vi "Variant to String.vi"(8 "error in (no error)":errorcluster, 10 "Variant":variant, 11 "Integer Value in":refnum<class "Integer Value.lvclass">) -> (0 "error out":errorcluster, 2 "String":string, 3 "Integer Value out":refnum<class "Integer Value.lvclass">)   [LabVIEW 2020, in "Composed Columns.lvlib" / "Integer Value.lvclass"]
uses:
  Integer Value.lvclass
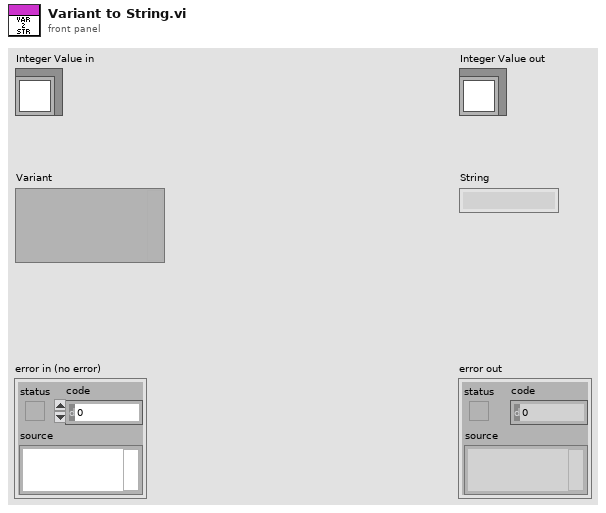
[diagram p1: front panel]
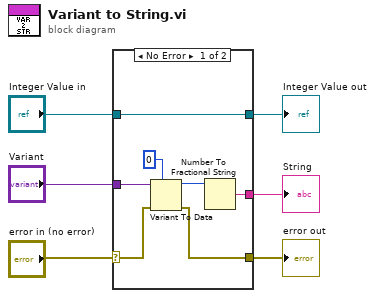
[diagram p0: block diagram]
diagram:
  n1 = case shown="No Error" "error in (no error)" {
    selector: "error in (no error)" -> [w9 w15]
    tunnel: "Integer Value in" -> [w7 w14]
    tunnel: [w8 w15] -> w1
    tunnel: [w7 w14] -> w3
    tunnel: "Variant" -> [w13 _]
    tunnel: [w10 _] -> w2
    frame No Error {
      n2 = Variant To Data(error in=w9, type=0, Variant=w13) -> (data=w11:i32, error out=w8:errorcluster)
      n3 = Number To Fractional String(number=w11) -> (F-format string=w10:string)  [unwired: 3 in]
    }
    frame Error {
    }
  }
  "error out" <- w1
  "Integer Value out" <- w3
  "String" <- w2
